vi "公式节点.vi"() -> ()   [LabVIEW 2017]
uses:
  <vilib>/express/express arith-compare/Formula/XNode/ExpressFormulaBlockNode.xnode
panel:
  out "波形图 2":dbl[][](graph)
  in  "b":dbl
  in  "m":dbl
  out "波形图":dbl[](graph)
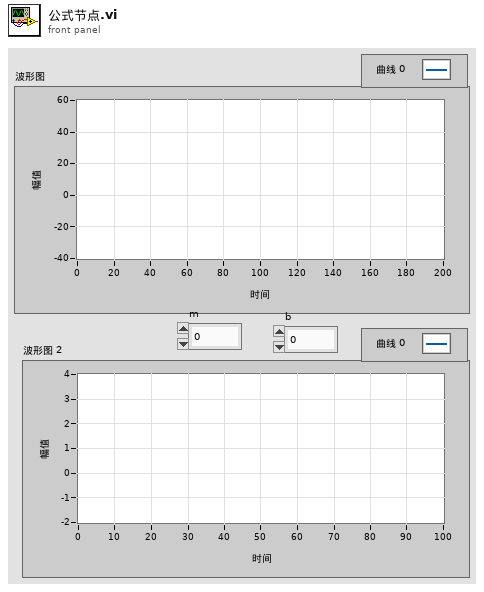
[diagram p1: front panel]
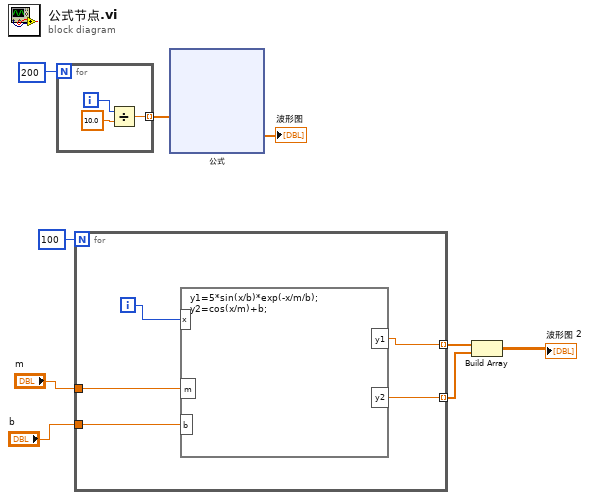
[diagram p0: block diagram]
diagram:
  n1 = for {
    N: 200 -> [_]
    tunnel: [w10] -> w8 mode=indexing
    i -> [w12]
    n2 = Divide(x=w12, y=10.0) -> (x/y=w10:dbl)
  }
  n3 = for {
    N: 100 -> [_]
    tunnel: "m" -> [w16]
    tunnel: "b" -> [w15]
    tunnel: [w14] -> w3 mode=indexing
    tunnel: [w13] -> w2 mode=indexing
    i -> [w17]
    n4 = formula code="y1=5*sin(x/b)*exp(-x/m/b);\ny2=cos(x/m)+b;"("x"=w17, "m"=w16, "b"=w15) -> ("y1"=w13:dbl, "y2"=w14:dbl)
  }
  n5 = xnode "公式"("X"=w8) -> ("结果"=→"波形图":dbl[])  [unwired: 1 in, 1 out]
  n6 = Build Array(w2, w3) -> (→"波形图 2":dbl[][])
